vi "SeCrTs-RT_Global_R.vi"() -> ()   [LabVIEW 2022 SP3]
panel:
  in  "Reader CS":refnum<k21>
  in  "Writer CS":refnum<k21>
  out "Connected?":bool
  out "Start daq":bool
  in  "RT Writer Stream_DD":refnum<k21>
  in  "RT Writer Stream_D":refnum<k21>
  in  "Lconnection ID":refnum<k5>
  in  "Aconnection ID":refnum<k5>
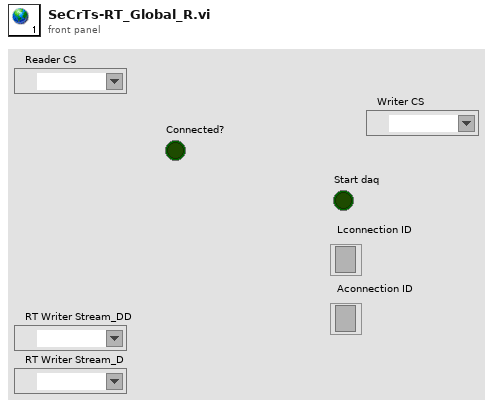
[diagram p1: front panel]
diagram:
